vi "Make Config File Header.vi"(0 "VISA resource name":refnum<visa-resource-name>, 11 "error in (no error)":errorcluster) -> (4 "VISA resource name out":refnum<visa-resource-name>, 6 "Result":string, 15 "error out":errorcluster)   [LabVIEW 2020, in "Yokogawa GX Series.lvlib"]
doc: "This VI sets the alarm hysteresis for <B>DX1000/DX2000 series</B>.\nThis VI can be used on Basic Setting Mode at the <B>Set Execution Mode.VI</B>.\n\nAlarm settings on computation channels can be specified on models with the /M1 or /PM1 math option.\nAlarm settings on external input channels can be specified on models with the /MC1 external input channel option."
uses:
  <instrlib>/Yokogawa GX Series/Yokogawa GX Series.lvlib
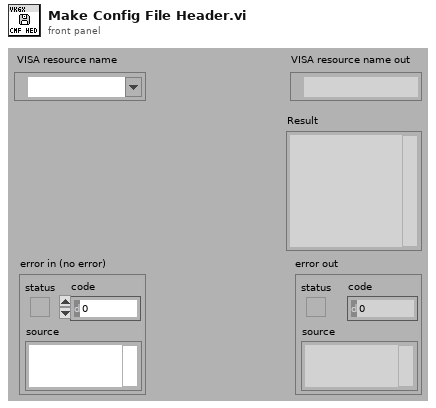
[diagram p1: front panel]
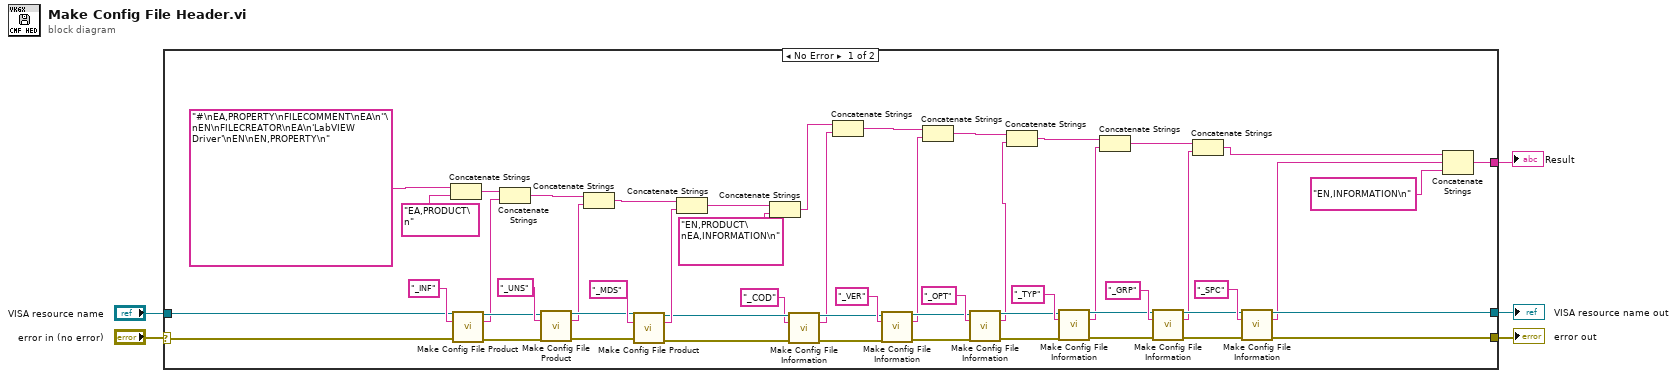
[diagram p0: block diagram]
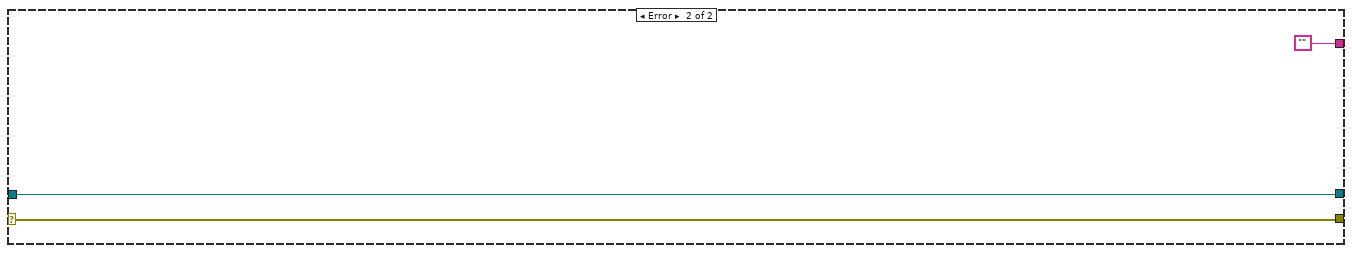
[diagram p2: hidden frame]
diagram:
  n1 = case shown="No Error" "error in (no error)" {
    selector: "error in (no error)" -> [w6 w59]
    tunnel: [w13 w60] -> w5
    tunnel: [w12 w59] -> w4
    tunnel: [w9 ""] -> w3
    tunnel: "VISA resource name" -> [w7 w60]
    frame No Error {
      n2 = Concatenate Strings("#\nEA,PROPERTY\nFILECOMMENT\nEA\n''\nEN\nFILECREATOR\nEA\n'LabVIEW Driver'\nEN\nEN,PROPERTY\n", "EA,PRODUCT\n") -> (w49:string)
      n3 = call <instrlib>:"Make Config File Product.vi"("VISA resource name"=w7, "Command (\"\")"="_INF", "error in (no error)"=w6) -> ("VISA resource name out"=w55:refnum<visa-resource-name>, "Result"=w48:string, "error out"=w54:errorcluster)  [unwired: 10 in]
      n4 = Concatenate Strings(w49, w48) -> (w47:string)
      n5 = call <instrlib>:"Make Config File Product.vi"("VISA resource name"=w55, "Command (\"\")"="_UNS", "error in (no error)"=w54) -> ("VISA resource name out"=w53:refnum<visa-resource-name>, "Result"=w46:string, "error out"=w52:errorcluster)  [unwired: 10 in]
      n6 = Concatenate Strings(w47, w46) -> (w45:string)
      n7 = call <instrlib>:"Make Config File Product.vi"("VISA resource name"=w53, "Command (\"\")"="_MDS", "error in (no error)"=w52) -> ("VISA resource name out"=w41:refnum<visa-resource-name>, "Result"=w44:string, "error out"=w40:errorcluster)  [unwired: 10 in]
      n8 = Concatenate Strings(w45, w44) -> (w42:string)
      n9 = Concatenate Strings(w42, "EN,PRODUCT\nEA,INFORMATION\n") -> (w20:string)
      n10 = call <instrlib>:"Make Config File Information.vi"("VISA resource name"=w41, "Command (\"\")"="_COD", "error in (no error)"=w40) -> ("VISA resource name out"=w33:refnum<visa-resource-name>, "Result"=w19:string, "error out"=w32:errorcluster)  [unwired: 10 in]
      n11 = Concatenate Strings(w20, w19) -> (w23:string)
      n12 = call <instrlib>:"Make Config File Information.vi"("VISA resource name"=w33, "Command (\"\")"="_VER", "error in (no error)"=w32) -> ("VISA resource name out"=w31:refnum<visa-resource-name>, "Result"=w18:string, "error out"=w30:errorcluster)  [unwired: 10 in]
      n13 = Concatenate Strings(w23, w18) -> (w22:string)
      n14 = call <instrlib>:"Make Config File Information.vi"("VISA resource name"=w31, "Command (\"\")"="_OPT", "error in (no error)"=w30) -> ("VISA resource name out"=w29:refnum<visa-resource-name>, "Result"=w17:string, "error out"=w28:errorcluster)  [unwired: 10 in]
      n15 = Concatenate Strings(w22, w17) -> (w21:string)
      n16 = call <instrlib>:"Make Config File Information.vi"("VISA resource name"=w29, "Command (\"\")"="_TYP", "error in (no error)"=w28) -> ("VISA resource name out"=w27:refnum<visa-resource-name>, "Result"=w16:string, "error out"=w26:errorcluster)  [unwired: 10 in]
      n17 = Concatenate Strings(w21, w16) -> (w15:string)
      n18 = call <instrlib>:"Make Config File Information.vi"("VISA resource name"=w27, "Command (\"\")"="_GRP", "error in (no error)"=w26) -> ("VISA resource name out"=w25:refnum<visa-resource-name>, "Result"=w14:string, "error out"=w24:errorcluster)  [unwired: 10 in]
      n19 = Concatenate Strings(w15, w14) -> (w10:string)
      n20 = call <instrlib>:"Make Config File Information.vi"("VISA resource name"=w25, "Command (\"\")"="_SPC", "error in (no error)"=w24) -> ("VISA resource name out"=w13:refnum<visa-resource-name>, "Result"=w11:string, "error out"=w12:errorcluster)  [unwired: 10 in]
      n21 = Concatenate Strings(w10, w11, "EN,INFORMATION\n") -> (w9:string)
    }
    frame Error {
    }
  }
  "error out" <- w4
  "VISA resource name out" <- w5
  "Result" <- w3
